vi "Autonomous State Machine Tote.vi"   [LabVIEW 2014]
doc: "This VI is called when autonomous begins, and will automatically be terminated when autonomous ends. You can carry out timed or sensor driven robot movement independently without needing to return to the caller."
uses:
  <vilib>/Rock Robotics/WPI/RobotDrive/WPI_RobotDriveGetSetRefNum.vi
panel:
  # "Be sure to right-click and choose Data Operations>>Make Current Value default if you want to save the array values with the VI"
types:
  T1 = typedef "WPI_MotorControlDeviceRef.ctl" = cluster{"DeviceStatus":errorcluster, "Type":T2, "PWM":cluster{"Controller":T3, "PWM Channel":T4, "DeadBand":T5}, "CAN":cluster{"Device Number":u8, "Control Mode":T6, "Semaphore":T7, "Max Vout":dbl, "TalonSRX Control Mode":T8}, "Invert":bool, "TransformRef":T9, "InvTransformRef":T9}
  T2 = typedef "WPI_MotorControlType.ctl" = enum16{"PWM", "CAN", "CANTalonSRX"}
  T3 = typedef "FPGA_TypedefDigitalModule.ctl" = enum16{"Controller 1"}
  T4 = typedef "FPGA_DIOPWMChannel.ctl" = enum8{"PWM 0", "PWM 1", "PWM 2", "PWM 3", "PWM 4", "PWM 5", "PWM 6", "PWM 7", "PWM 8", "PWM 9", "PWM MXP 0", "PWM MXP 1", "PWM MXP 2", "PWM MXP 3", "PWM MXP 4", "PWM MXP 5", "PWM MXP 6", "PWM MXP 7", "PWM MXP 8", "PWM MXP 9", "Invalid"}
  T5 = typedef "WPI_PWMDeadband.ctl" = cluster{"Name":string, "maxPositivePwm":i32, "minPositivePwm":i32, "centerPwm":i32, "maxNegativePwm":i32, "minNegativePwm":i32, "angularRange":u16}
  T6 = typedef "WPI_CANJaguar_ControlMode.ctl" = enum8{"Percent VBus", "Current", "Speed", "Position", "Voltage"}
  T7 = typedef "Semaphore RefNum" = refnum<k1>
  T8 = typedef "WPI_CANTalonSRX_APIControlMode.ctl" = enum8{"Percent VBus", "Speed", "Position", "Slave", "Unchanged / Invalid"}
  T9 = typedef "WPI_PWMTransform_ConPane.ctl" = refnum<vi>
  T10 = typedef "WPI_CANTalonSRX_GlobalStatus.ctl" = cluster{"Applied Throttle":dbl, "Module Enabled":bool, "CAN Error":errorcluster, "Closed Loop Error":dbl, "Forward Limit Switch Closed":bool, "Reverse Limit Switch Closed":bool, "Sensor Position":dbl, "Sensor Velocity":dbl, "Current":dbl, "Sticky Fault - Over Temp":bool, "Sticky Fault - Under Voltage":bool, "Sticky Fault - Forward Limit":bool, "Sticky Fault - Reverse Limit":bool, "Sticky Fault - Forward Soft Limit":bool, "Sticky Fault - Reverse Soft Limit":bool, "Brake is Enabled":bool, "Encoder Position":dbl, "Encoder Velocity":dbl, "Encoder Index Count":dbl, "Encoder A Pin State":bool, "Encoder B Pin State":bool, "Encoder Index Pin State":bool, "Analog In":dbl, "Analog In Velocity":dbl, "Temperature (C)":dbl, "Battery Voltage":dbl}
  T11 = typedef "WPI_EncoderDevRef.ctl" = cluster{"DevStatus":errorcluster, "EncoderIndex":T12, "CounterIndex":T13, "DistancePerCount":dbl, "Decoding Type":T14}
  T12 = typedef "FPGA_EncoderIdx.ctl" = enum8{"Enc 0", "Enc 1", "Enc 2", "Enc 3", "Enc 4", "Enc 5", "Enc 6", "Enc 7", "Invalid"}
  T13 = typedef "FPGA_CounterCtrSystemIndex.ctl" = enum8{"Ctr 0", "Ctr 1", "Ctr 2", "Ctr 3", "Ctr 4", "Ctr 5", "Ctr 6", "Ctr 7", "Invalid"}
  T14 = typedef "WPI_EncoderType.ctl" = enum16{"1x", "2x", "4x"}
  T15 = typedef "WPI_RobotDriveDevRef.ctl" = cluster{"DevStatus":errorcluster, "Motors[]":T1[], "Square Inputs":bool, "Max Output":dbl}
  T16 = typedef "WPI_SwitchDevRef.ctl" = cluster{"DevStatus":errorcluster, "DIO Channel":T17, "Controller":T3, "CntIndex":T13, "Normally Closed":bool}
  T17 = typedef "FPGA_DIOChannel.ctl" = enum8{"DIO 0", "DIO 1", "DIO 2", "DIO 3", "DIO 4", "DIO 5", "DIO 6", "DIO 7", "DIO 8", "DIO 9", "DIO MXP 0", "DIO MXP 1", "DIO MXP 2", "DIO MXP 3", "DIO MXP 4", "DIO MXP 5", "DIO MXP 6", "DIO MXP 7", "DIO MXP 8", "DIO MXP 9", "DIO MXP 10", "DIO MXP 11", "DIO MXP 12", "DIO MXP 13", "DIO MXP 14", "DIO MXP 15", "Invalid"}
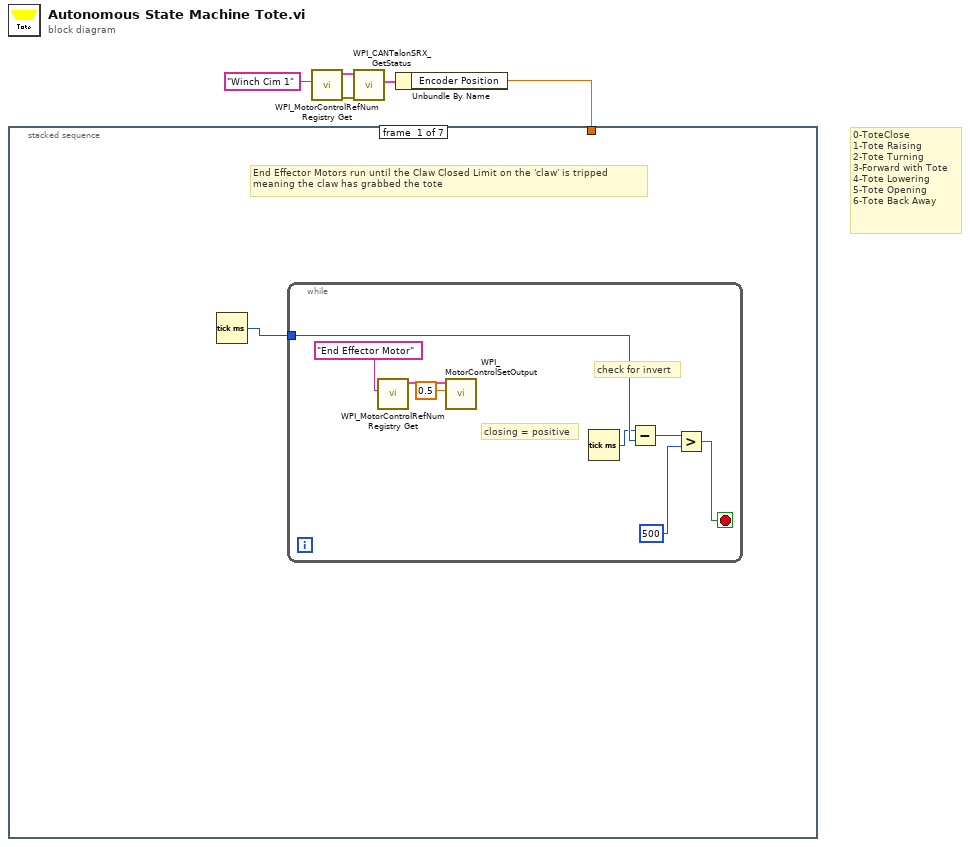
[diagram p0: block diagram]
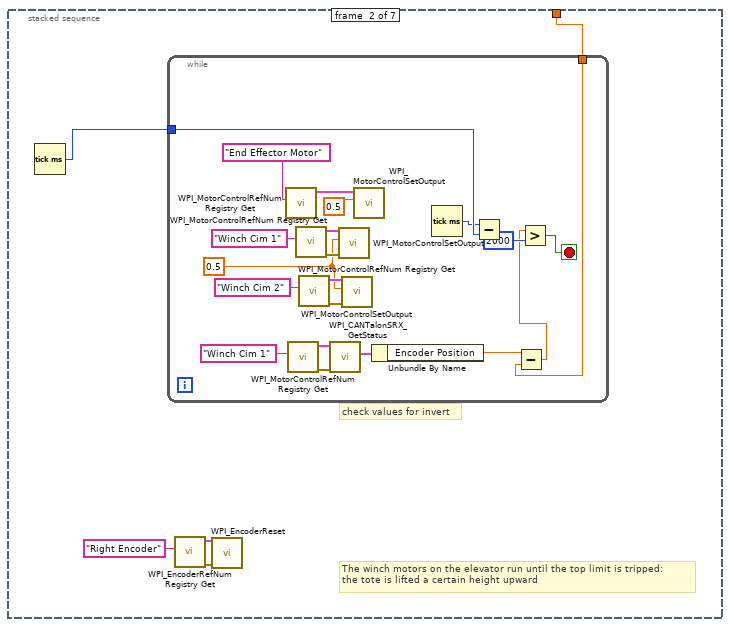
[diagram p2: hidden frame]
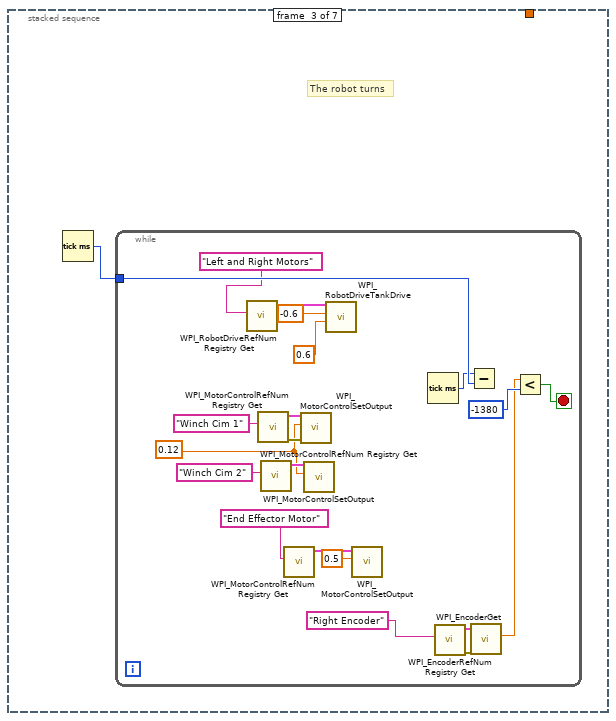
[diagram p3: hidden frame]
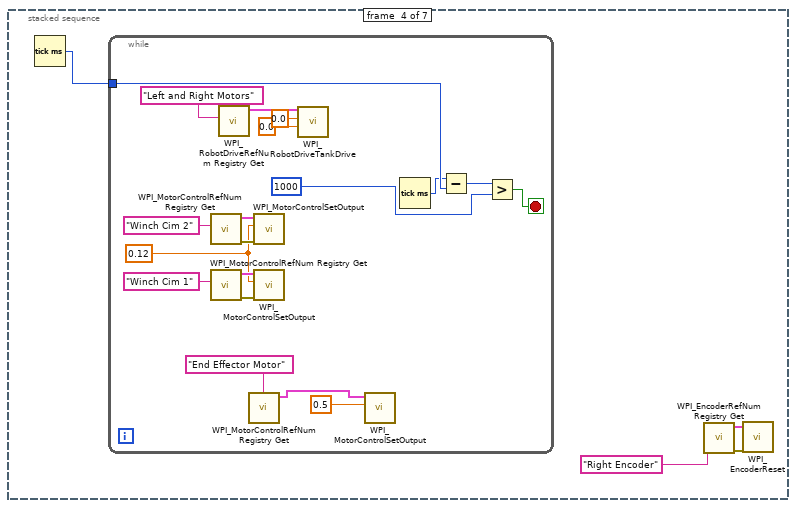
[diagram p4: hidden frame]
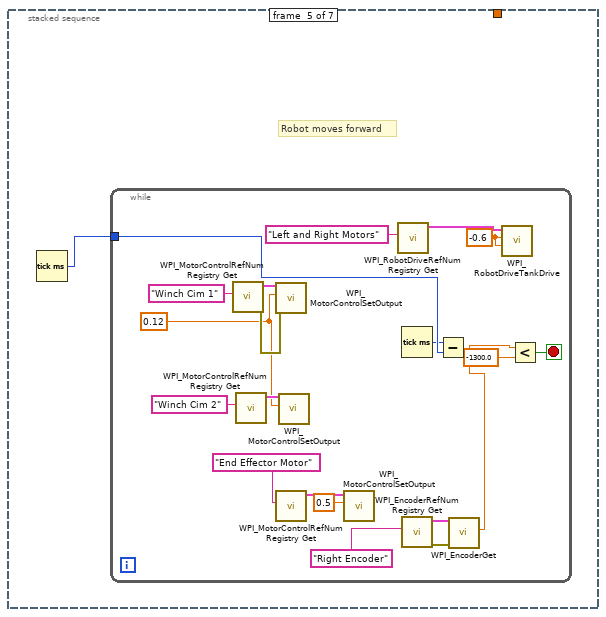
[diagram p5: hidden frame]
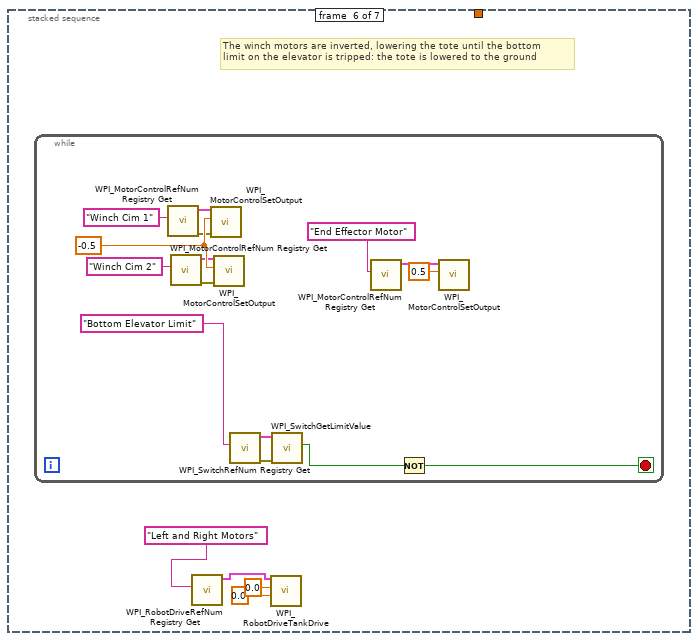
[diagram p6: hidden frame]
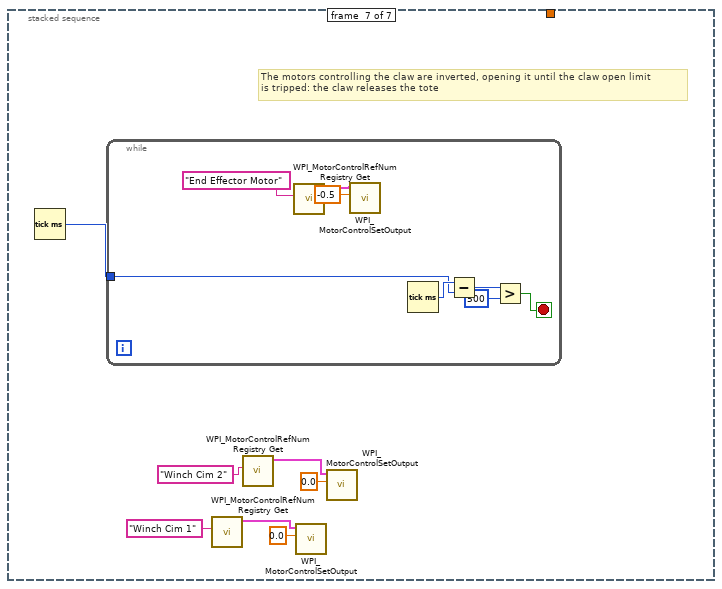
[diagram p7: hidden frame]
diagram:
  # "0-ToteClose\n1-Tote Raising\n2-Tote Turning\n3-Forward with Tote\n4-Tote Lowering\n5-Tote Opening\n6-Tote Back Away"
  n1 = call <vilib>:"WPI_MotorControlRefNum Registry Get.vi"("refnum name"="Winch Cim 1") -> ("error out"=w5:errorcluster, "MotorControlDevRef"=w4:T1)  [unwired: 9 in]
  n2 = call <vilib>:"WPI_CANTalonSRX_GetStatus.vi"("error in (no error)"=w5, "CAN Talon SRX Ref"=w4) -> ("Talon SRX Status"=w2:T10)  [unwired: 7 in, 2 out]
  n3 = Unbundle By Name(w2) -> ("Encoder Position"=w1:dbl)
  n4 = stacked-sequence {
    tunnel: w1 -> [_ w18 _ _ _ _ _]
    frame #0 {
      # "End Effector Motors run until the Claw Closed Limit on the 'claw' is tripped\nmeaning the claw has grabbed the tote"
      n5 = Tick Count (ms)() -> (millisecond timer value=w6:u32)
      n6 = while {
        tunnel: w6 -> [w11]
        stop <- w12 stop-if-true
        # "closing = positive"
        # "check for invert"
        n7 = call <vilib>:"WPI_MotorControlRefNum Registry Get.vi"("refnum name"="End Effector Motor") -> ("MotorControlDevRef"=w7:T1)  [unwired: 9 in, 1 out]
        n8 = call <vilib>:"WPI_MotorControlSetOutput.vi"("Output"=0.5, "MotorControlDevRef"=w7) -> ()  [unwired: 7 in, 3 out]
        n9 = Tick Count (ms)() -> (millisecond timer value=w10:u32)
        n10 = Subtract(x=w10, y=w11) -> (x-y=w14:u32)
        n11 = Greater?(x=w14, y=u32 500) -> (0:w12:bool)
      }
    }
    frame #1 {
      # "The winch motors on the elevator run until the top limit is tripped: \nthe tote is lifted a certain height upward"
      # "check values for invert"
      n12 = Tick Count (ms)() -> (millisecond timer value=w19:u32)
      n13 = while {
        tunnel: w19 -> [w38]
        tunnel: w18 -> [w21]
        stop <- w39 stop-if-true
        w30 = 0.5
        n14 = call <vilib>:"WPI_MotorControlRefNum Registry Get.vi"("refnum name"="End Effector Motor") -> ("MotorControlDevRef"=w29:T1)  [unwired: 9 in, 1 out]
        n15 = call <vilib>:"WPI_MotorControlRefNum Registry Get.vi"("refnum name"="Winch Cim 1") -> ("error out"=w26:errorcluster, "MotorControlDevRef"=w25:T1)  [unwired: 9 in]
        n16 = call <vilib>:"WPI_MotorControlRefNum Registry Get.vi"("refnum name"="Winch Cim 1") -> ("error out"=w35:errorcluster, "MotorControlDevRef"=w34:T1)  [unwired: 9 in]
        n17 = call <vilib>:"WPI_MotorControlRefNum Registry Get.vi"("refnum name"="Winch Cim 2") -> ("error out"=w32:errorcluster, "MotorControlDevRef"=w31:T1)  [unwired: 9 in]
        n18 = call <vilib>:"WPI_CANTalonSRX_GetStatus.vi"("error in (no error)"=w26, "CAN Talon SRX Ref"=w25) -> ("Talon SRX Status"=w23:T10)  [unwired: 7 in, 2 out]
        n19 = call <vilib>:"WPI_MotorControlSetOutput.vi"("error in (no error)"=w35, "Output"=w30, "MotorControlDevRef"=w34) -> ()  [unwired: 6 in, 3 out]
        n20 = call <vilib>:"WPI_MotorControlSetOutput.vi"("error in (no error)"=w32, "Output"=w30, "MotorControlDevRef"=w31) -> ()  [unwired: 6 in, 3 out]
        n21 = call <vilib>:"WPI_MotorControlSetOutput.vi"("Output"=0.5, "MotorControlDevRef"=w29) -> ()  [unwired: 7 in, 3 out]
        n22 = Unbundle By Name(w23) -> ("Encoder Position"=w22:dbl)
        n23 = Tick Count (ms)() -> (millisecond timer value=w37:u32)
        n24 = Subtract(x=w37, y=w38) -> ()  [unwired: 1 out]
        n25 = Subtract(x=w22, y=w21) -> (x-y=w20:dbl)
        n26 = Greater?(x=w20, y=u32 2000) -> (0:w39:bool)
      }
      n27 = call <vilib>:"WPI_EncoderRefNum Registry Get.vi"("refnum name"="Right Encoder") -> ("error out"=w17:errorcluster, "EncoderDevRef"=w16:T11)  [unwired: 9 in]
      n28 = call <vilib>:"WPI_EncoderReset.vi"("error in (no error)"=w17, "EncoderDevRef"=w16) -> ()  [unwired: 8 in, 2 out]
    }
    frame #2 {
      # "The robot turns"
      n29 = Tick Count (ms)() -> (millisecond timer value=w41:u32)
      n30 = while {
        tunnel: w41 -> [w60]
        stop <- w61 stop-if-true
        w50 = 0.12
        n31 = call <vilib>:"WPI_RobotDriveRefNum Registry Get.vi"("refnum name"="Left and Right Motors") -> ("RobotDriveDevRef"=w58:T15)  [unwired: 9 in, 1 out]
        n32 = call <vilib>:"WPI_MotorControlRefNum Registry Get.vi"("refnum name"="Winch Cim 1") -> ("error out"=w53:errorcluster, "MotorControlDevRef"=w49:T1)  [unwired: 9 in]
        n33 = call <vilib>:"WPI_MotorControlRefNum Registry Get.vi"("refnum name"="Winch Cim 2") -> ("MotorControlDevRef"=w51:T1)  [unwired: 9 in, 1 out]
        n34 = call <vilib>:"WPI_MotorControlRefNum Registry Get.vi"("refnum name"="End Effector Motor") -> ("MotorControlDevRef"=w46:T1)  [unwired: 9 in, 1 out]
        n35 = call <vilib>:"WPI_MotorControlSetOutput.vi"("error in (no error)"=w53, "Output"=w50, "MotorControlDevRef"=w49) -> ()  [unwired: 6 in, 3 out]
        n36 = call <vilib>:"WPI_MotorControlSetOutput.vi"("Output"=w50, "MotorControlDevRef"=w51) -> ()  [unwired: 7 in, 3 out]
        n37 = call <vilib>:"WPI_RobotDriveTankDrive.vi"("Right axis value"=0.6, "Left axis value"=-0.6, "RobotDriveDevRef"=w58) -> ()  [unwired: 6 in, 3 out]
        n38 = call <vilib>:"WPI_MotorControlSetOutput.vi"("Output"=0.5, "MotorControlDevRef"=w46) -> ()  [unwired: 7 in, 3 out]
        n39 = Tick Count (ms)() -> (millisecond timer value=w59:u32)
        n40 = call <vilib>:"WPI_EncoderRefNum Registry Get.vi"("refnum name"="Right Encoder") -> ("error out"=w45:errorcluster, "EncoderDevRef"=w44:T11)  [unwired: 9 in]
        n41 = Subtract(x=w59, y=w60) -> ()  [unwired: 1 out]
        n42 = call <vilib>:"WPI_EncoderGet.vi"("error in (no error)"=w45, "EncoderDevRef"=w44) -> ("Distance"=w42:dbl)  [unwired: 4 in, 5 out]
        n43 = Less?(x=w42, y=-1380) -> (x < y?=w61:bool)
      }
    }
    frame #3 {
      n44 = Tick Count (ms)() -> (millisecond timer value=w66:u32)
      n45 = while {
        tunnel: w66 -> [w83]
        stop <- w84 stop-if-true
        w70 = 0.12
        n46 = call <vilib>:"WPI_MotorControlRefNum Registry Get.vi"("refnum name"="Winch Cim 2") -> ("error out"=w72:errorcluster, "MotorControlDevRef"=w71:T1)  [unwired: 9 in]
        n47 = call <vilib>:"WPI_MotorControlRefNum Registry Get.vi"("refnum name"="Winch Cim 1") -> ("error out"=w75:errorcluster, "MotorControlDevRef"=w74:T1)  [unwired: 9 in]
        n48 = call <vilib>:"WPI_RobotDriveRefNum Registry Get.vi"("refnum name"="Left and Right Motors") -> ("RobotDriveDevRef"=w81:T15)  [unwired: 9 in, 1 out]
        n49 = call <vilib>:"WPI_MotorControlRefNum Registry Get.vi"("refnum name"="End Effector Motor") -> ("MotorControlDevRef"=w67:T1)  [unwired: 9 in, 1 out]
        n50 = call <vilib>:"WPI_MotorControlSetOutput.vi"("error in (no error)"=w72, "Output"=w70, "MotorControlDevRef"=w71) -> ()  [unwired: 6 in, 3 out]
        n51 = call <vilib>:"WPI_MotorControlSetOutput.vi"("error in (no error)"=w75, "Output"=w70, "MotorControlDevRef"=w74) -> ()  [unwired: 6 in, 3 out]
        n52 = call <vilib>:"WPI_RobotDriveTankDrive.vi"("Right axis value"=0.0, "Left axis value"=0.0, "RobotDriveDevRef"=w81) -> ()  [unwired: 6 in, 3 out]
        n53 = call <vilib>:"WPI_MotorControlSetOutput.vi"("Output"=0.5, "MotorControlDevRef"=w67) -> ()  [unwired: 7 in, 3 out]
        n54 = Tick Count (ms)() -> (millisecond timer value=w82:u32)
        n55 = Subtract(x=w82, y=w83) -> (x-y=w85:u32)
        n56 = Greater?(x=w85, y=1000) -> (0:w84:bool)
      }
      n57 = call <vilib>:"WPI_EncoderRefNum Registry Get.vi"("refnum name"="Right Encoder") -> ("error out"=w65:errorcluster, "EncoderDevRef"=w64:T11)  [unwired: 9 in]
      n58 = call <vilib>:"WPI_EncoderReset.vi"("error in (no error)"=w65, "EncoderDevRef"=w64) -> ()  [unwired: 8 in, 2 out]
    }
    frame #4 {
      # "Robot moves forward"
      n59 = Tick Count (ms)() -> (millisecond timer value=w86:u32)
      n60 = while {
        tunnel: w86 -> [w105]
        stop <- w106 stop-if-true
        w96 = 0.12
        w101 = -0.6 ("Left axis value")
        n61 = call <vilib>:"WPI_MotorControlRefNum Registry Get.vi"("refnum name"="Winch Cim 1") -> ("error out"=w99:errorcluster, "MotorControlDevRef"=w95:T1)  [unwired: 9 in]
        n62 = call <vilib>:"WPI_MotorControlRefNum Registry Get.vi"("refnum name"="Winch Cim 2") -> ("MotorControlDevRef"=w97:T1)  [unwired: 9 in, 1 out]
        n63 = call <vilib>:"WPI_MotorControlSetOutput.vi"("error in (no error)"=w99, "Output"=w96, "MotorControlDevRef"=w95) -> ()  [unwired: 6 in, 3 out]
        n64 = call <vilib>:"WPI_MotorControlRefNum Registry Get.vi"("refnum name"="End Effector Motor") -> ("MotorControlDevRef"=w92:T1)  [unwired: 9 in, 1 out]
        n65 = call <vilib>:"WPI_MotorControlSetOutput.vi"("Output"=w96, "MotorControlDevRef"=w97) -> ()  [unwired: 7 in, 3 out]
        n66 = call <vilib>:"WPI_MotorControlSetOutput.vi"("Output"=0.5, "MotorControlDevRef"=w92) -> ()  [unwired: 7 in, 3 out]
        n67 = call <vilib>:"WPI_RobotDriveRefNum Registry Get.vi"("refnum name"="Left and Right Motors") -> ("RobotDriveDevRef"=w103:T15)  [unwired: 9 in, 1 out]
        n68 = Tick Count (ms)() -> (millisecond timer value=w104:u32)
        n69 = call <vilib>:"WPI_EncoderRefNum Registry Get.vi"("refnum name"="Right Encoder") -> ("error out"=w90:errorcluster, "EncoderDevRef"=w89:T11)  [unwired: 9 in]
        n70 = Subtract(x=w104, y=w105) -> ()  [unwired: 1 out]
        n71 = call <vilib>:"WPI_EncoderGet.vi"("error in (no error)"=w90, "EncoderDevRef"=w89) -> ("Distance"=w88:dbl)  [unwired: 4 in, 5 out]
        n72 = call <vilib>:"WPI_RobotDriveTankDrive.vi"("Right axis value"=w101, "Left axis value"=w101, "RobotDriveDevRef"=w103) -> ()  [unwired: 6 in, 3 out]
        n73 = Less?(x=w88, y=-1300.0) -> (x < y?=w106:bool)
      }
    }
    frame #5 {
      # "The winch motors are inverted, lowering the tote until the bottom \nlimit on the elevator is tripped: the tote is lowered to the ground"
      n74 = while {
        stop <- w114 stop-if-true
        w125 = -0.5
        n75 = call <vilib>:"WPI_MotorControlRefNum Registry Get.vi"("refnum name"="Winch Cim 1") -> ("error out"=w120:errorcluster, "MotorControlDevRef"=w121:T1)  [unwired: 9 in]
        n76 = call <vilib>:"WPI_MotorControlRefNum Registry Get.vi"("refnum name"="Winch Cim 2") -> ("error out"=w123:errorcluster, "MotorControlDevRef"=w124:T1)  [unwired: 9 in]
        n77 = call <vilib>:"WPI_MotorControlSetOutput.vi"("error in (no error)"=w120, "Output"=w125, "MotorControlDevRef"=w121) -> ()  [unwired: 6 in, 3 out]
        n78 = call <vilib>:"WPI_MotorControlSetOutput.vi"("error in (no error)"=w123, "Output"=w125, "MotorControlDevRef"=w124) -> ()  [unwired: 6 in, 3 out]
        n79 = call <vilib>:"WPI_SwitchRefNum Registry Get.vi"("refnum name"="Bottom Elevator Limit") -> ("error out"=w118:errorcluster, "SwitchDevRef"=w117:T16)  [unwired: 9 in]
        n80 = call <vilib>:"WPI_SwitchGetLimitValue.vi"("error in (no error)"=w118, "SwitchDevRef"=w117) -> ("Switch Pressed"=w115:bool)  [unwired: 7 in, 2 out]
        n81 = call <vilib>:"WPI_MotorControlRefNum Registry Get.vi"("refnum name"="End Effector Motor") -> ("MotorControlDevRef"=w111:T1)  [unwired: 9 in, 1 out]
        n82 = Not(x=w115) -> (.not. x?=w114:bool)
        n83 = call <vilib>:"WPI_MotorControlSetOutput.vi"("Output"=0.5, "MotorControlDevRef"=w111) -> ()  [unwired: 7 in, 3 out]
      }
      n84 = call <vilib>:"WPI_RobotDriveRefNum Registry Get.vi"("refnum name"="Left and Right Motors") -> ("RobotDriveDevRef"=w110:T15)  [unwired: 9 in, 1 out]
      n85 = call <vilib>:"WPI_RobotDriveTankDrive.vi"("Right axis value"=0.0, "Left axis value"=0.0, "RobotDriveDevRef"=w110) -> ()  [unwired: 6 in, 3 out]
    }
    frame #6 {
      # "The motors controlling the claw are inverted, opening it until the claw open limit\nis tripped: the claw releases the tote"
      n86 = Tick Count (ms)() -> (millisecond timer value=w132:u32)
      n87 = while {
        tunnel: w132 -> [w133]
        stop <- w138 stop-if-true
        n88 = call <vilib>:"WPI_MotorControlRefNum Registry Get.vi"("refnum name"="End Effector Motor") -> ("MotorControlDevRef"=w135:T1)  [unwired: 9 in, 1 out]
        n89 = call <vilib>:"WPI_MotorControlSetOutput.vi"("Output"=-0.5, "MotorControlDevRef"=w135) -> ()  [unwired: 7 in, 3 out]
        n90 = Tick Count (ms)() -> (millisecond timer value=w137:u32)
        n91 = Subtract(x=w137, y=w133) -> (x-y=w140:u32)
        n92 = Greater?(x=w140, y=u32 500) -> (0:w138:bool)
      }
      n93 = call <vilib>:"WPI_MotorControlRefNum Registry Get.vi"("refnum name"="Winch Cim 1") -> ("MotorControlDevRef"=w127:T1)  [unwired: 9 in, 1 out]
      n94 = call <vilib>:"WPI_MotorControlRefNum Registry Get.vi"("refnum name"="Winch Cim 2") -> ("MotorControlDevRef"=w130:T1)  [unwired: 9 in, 1 out]
      n95 = call <vilib>:"WPI_MotorControlSetOutput.vi"("Output"=0.0, "MotorControlDevRef"=w127) -> ()  [unwired: 7 in, 3 out]
      n96 = call <vilib>:"WPI_MotorControlSetOutput.vi"("Output"=0.0, "MotorControlDevRef"=w130) -> ()  [unwired: 7 in, 3 out]
    }
  }
